vi "myRIO_BRig_generic_pathExists_fast_pathInput.vi"(8 "input_error":errorcluster, 11 "input_filePath":path) -> (0 "output_error":errorcluster, 2 "output_Iexist":bool, 3 "output_filePath":path)   [LabVIEW 2014]
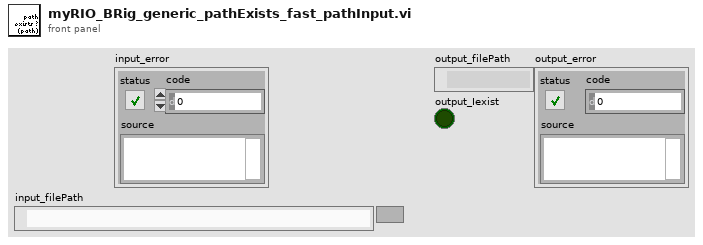
[diagram p1: front panel]
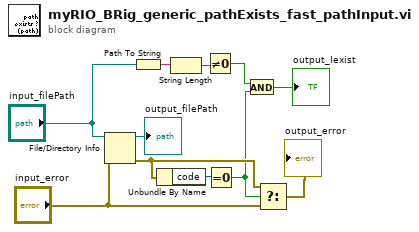
[diagram p0: block diagram]
diagram:
  n1 = File/Directory Info(path="input_filePath", error in="input_error") -> (path out=→"output_filePath":path, error out=w8:errorcluster)  [unwired: 5 out]
  n2 = Path To String(path="input_filePath") -> (string=w5:string)
  n3 = Unbundle By Name(w8) -> ("code"=w10:i32)
  n4 = String Length(string=w5) -> (length=w4:i32)
  n5 = Not Equal To 0?(x=w4) -> (x != 0?=w3:bool)
  n6 = Equal To 0?(x=w10) -> (x = 0?=w2:bool)
  n7 = And(x=w3, y=w2) -> (x .and. y?=→"output_Iexist":bool)
  n8 = Select(t=w8, s=w2, f="input_error") -> (s? t:f=→"output_error":errorcluster)
